vi "SCA Sample-Encoder conversion.vi"(6 "Step Window Radius":i16, 7 "Rollover Sample":i16, 9 "Encoder Offset":i16, 10 "Encoder Position":i16, 11 "Desired Sample":u8) -> (1 "Window limit 1":i16, 2 "Within Range?":bool, 3 "Encoder destination":i16, 4 "Window limit 2":i16, 5 "New move (encoder steps)":i16)   [LabVIEW 2016]
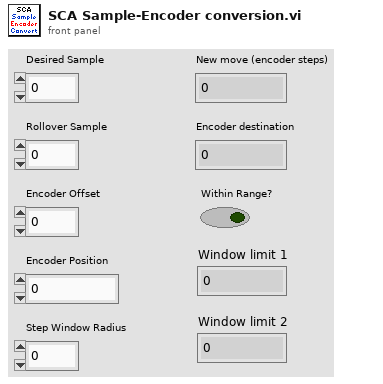
[diagram p1: front panel]
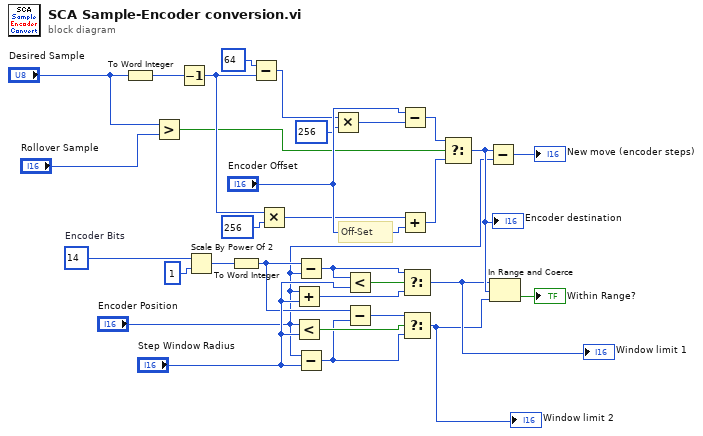
[diagram p0: block diagram]
diagram:
  w29 = i16 14  # Encoder Bits
  # "Off-Set"
  n1 = To Word Integer(number="Desired Sample") -> (16bit integer=w2:i16)
  n2 = Greater?(x="Desired Sample", y="Rollover Sample") -> (0:w23:bool)
  n3 = Decrement(x=w2) -> (x-1=w27:i16)
  n4 = Scale By Power Of 2(n=w29, x=u32 1) -> (x*2^n=w30:u32)
  n5 = To Word Integer(number=w30) -> (16bit integer=w4:i16)
  n6 = Subtract(x=i16 64, y=w27) -> (x-y=w21:i16)
  n7 = Multiply(x=w27, y=i16 256) -> (x*y=w15:i16)
  n8 = Add(x="Encoder Position", y="Step Window Radius") -> (x+y=w5:i16)
  n9 = Less?(x="Encoder Position", y="Step Window Radius") -> (x < y?=w11:bool)
  n10 = Subtract(x=w4, y="Encoder Position") -> (x-y=w6:i16)
  n11 = Subtract(x="Encoder Position", y="Step Window Radius") -> (x-y=w8:i16)
  n12 = Multiply(x=w21, y=i16 256) -> (x*y=w22:i16)
  n13 = Less?(x=w6, y="Step Window Radius") -> (x < y?=w7:bool)
  n14 = Subtract(x=w4, y=w8) -> (x-y=w10:i16)
  n15 = Subtract(x="Encoder Offset", y=w22) -> (x-y=w24:i16)
  n16 = Add(x=w15, y="Encoder Offset") -> (x+y=w25:i16)
  n17 = Select(t=w6, s=w7, f=w5) -> (s? t:f=w17:i16)
  "Window limit 1" <- w17
  n18 = Select(t=w10, s=w11, f=w8) -> (s? t:f=w16:i16)
  "Window limit 2" <- w16
  n19 = Select(t=w24, s=w23, f=w25) -> (s? t:f=w26:i16)
  "Encoder destination" <- w26
  n20 = Subtract(x=w26, y="Encoder Position") -> (x-y=→"New move (encoder steps)":i16)
  n21 = In Range and Coerce(upper limit=w17, x=w26, lower limit=w16) -> (In Range?=→"Within Range?":bool)  [unwired: 1 out]
